vi "Calculate Current or Voltage Values from Slew Rate.vi"(9 "Current/voltage slew rate":dbl, 10 "Current/voltage end point":dbl, 11 "Current/voltage start point":dbl) -> (2 "Source delays":dbl[](array[numeric]), 3 "Current/voltage values":dbl[](array[numeric]))   [LabVIEW 2021, in "PMIC Common.lvlib"]
uses:
  PMIC Common.lvlib
  <vilib>/Analysis/NI_AALBase.lvlib
  <vilib>/Analysis/1siggen.llb/Ramp Pattern by Samples.vi
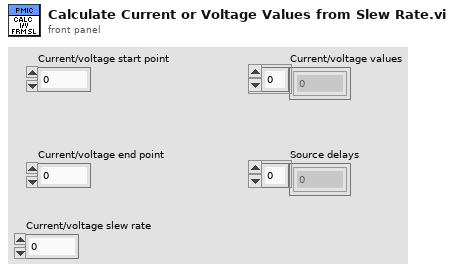
[diagram p1: front panel]
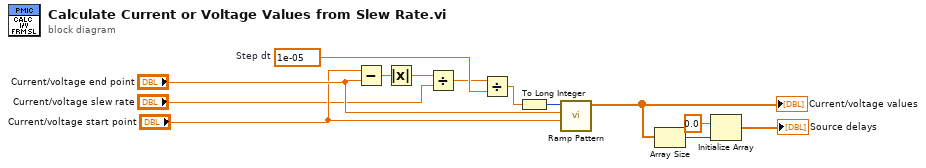
[diagram p0: block diagram]
diagram:
  w7 = 1e-05  # Step dt
  n1 = Subtract(x="Current/voltage start point", y="Current/voltage end point") -> (x-y=w1:dbl)
  n2 = Absolute Value(x=w1) -> (abs(x)=w2:dbl)
  n3 = Divide(x=w2, y="Current/voltage slew rate") -> (x/y=w3:dbl)
  n4 = Divide(x=w3, y=w7) -> (x/y=w4:dbl)
  n5 = To Long Integer(number=w4) -> (32bit integer=w8:i32)
  n6 = call-poly <vilib>:"Ramp Pattern.vi"("start"="Current/voltage start point", "end"="Current/voltage end point", "samples"=w8) -> ("Ramp Pattern"=w10:dbl[])  [unwired: 7 in, 1 out]
  "Current/voltage values" <- w10
  n7 = Array Size(array=w10) -> (size(s)=w6:i32)
  n8 = Initialize Array(0.0 ("element"), w6) -> (→"Source delays":dbl[])
